vi "DeviceSetNiAuthPasswordRequest_Parse.vi"(8 "error in (no error)":errorcluster, 11 "Message":T5) -> (0 "error out":errorcluster, 1 "Body":T1, 2 "Header":T3, 3 "DeviceSetNiAuthPasswordRequest":T2)   [LabVIEW 2017]
uses:
  <vilib>/addons/InsightCM/MessageBus/Base/controls/Message.ctl
  <vilib>/addons/InsightCM/MessageBus/Base/controls/MessageHeader.ctl
  <vilib>/addons/InsightCM/MessageBus/Base/controls/KeyValuePair.ctl
  <vilib>/addons/InsightCM/MessageBus/MessageLibrary/Device/controls/DeviceSetNiAuthPasswordRequest.ctl
  <vilib>/addons/InsightCM/MessageBus/MessageLibrary/Device/controls/DeviceSetNiAuthPasswordRequestBody.ctl
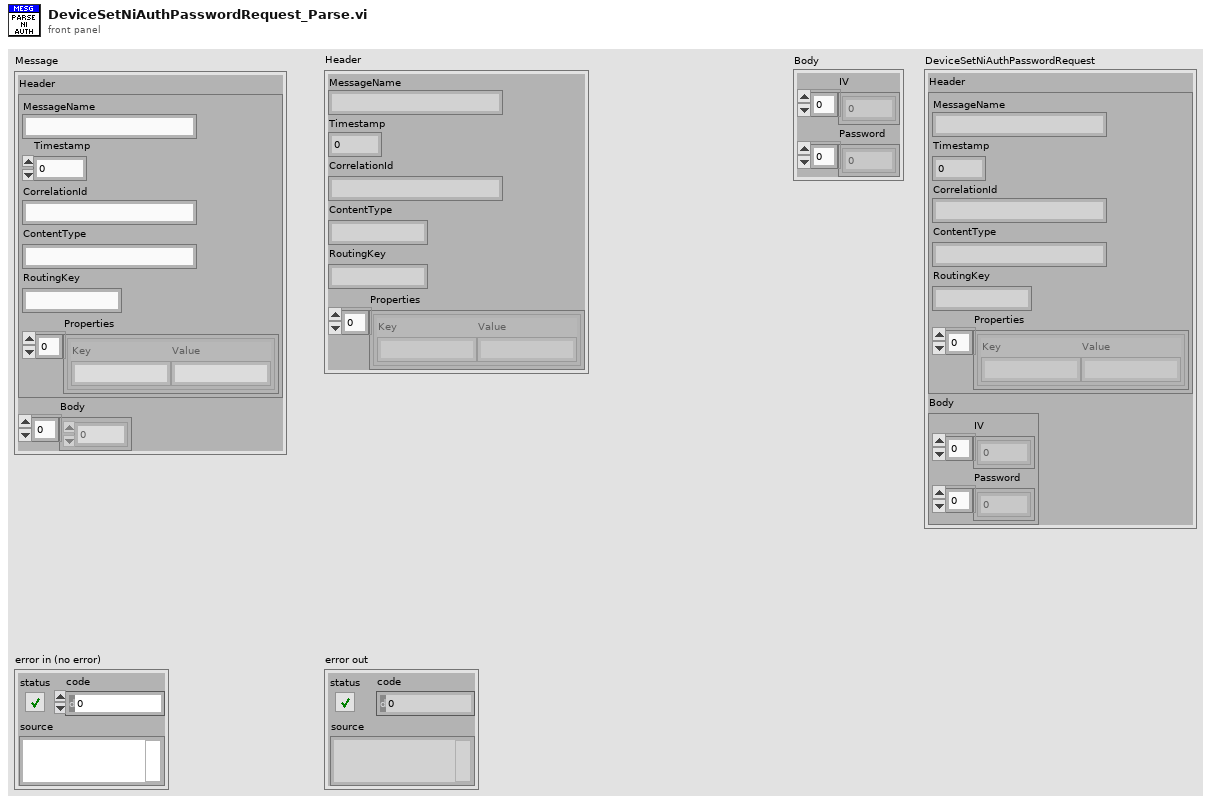
[diagram p1: front panel]
types:
  T1 = typedef "DeviceSetNiAuthPasswordRequestBody.ctl" = cluster{"IV":u8[], "Password":u8[]}
  T2 = typedef "DeviceSetNiAuthPasswordRequest.ctl" = cluster{"Header":T3, "Body":T1}
  T3 = typedef "MessageHeader.ctl" = cluster{"MessageName":string, "Timestamp":i64, "CorrelationId":string, "ContentType":string, "RoutingKey":string, "Properties":T4[]}
  T4 = typedef "KeyValuePair.ctl" = cluster{"Key":string, "Value":string}
  T5 = typedef "Message.ctl" = cluster{"Header":T3, "Body":u8[]}
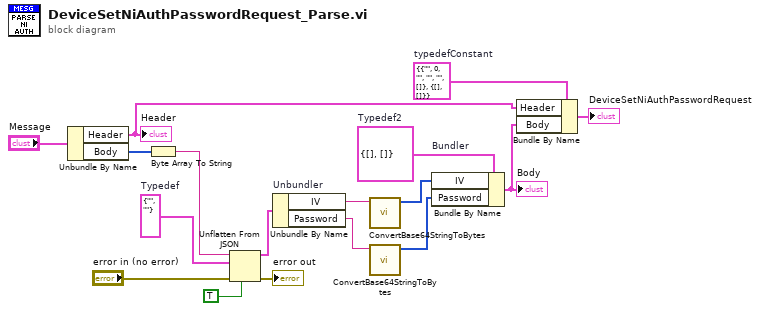
[diagram p0: block diagram]
diagram:
  w5 = T1 {"IV"=[], "Password"=[]}  # Typedef2
  w9 = T2 {"Header"={"MessageName"="", "Timestamp"=0, "CorrelationId"="", "ContentType"="", "RoutingKey"="", "Properties"=[]}, "Body"={"IV"=[], "Password"=[]}}  # typedefConstant
  w13 = cluster{"IV":string, "Password":string} {"IV"="", "Password"=""}  # Typedef
  n1 = Unbundle By Name("Message") -> ("Header"=w15:T3, "Body"=w7:u8[])
  "Header" <- w15
  n2 = Byte Array To String(unsigned byte array=w7) -> (string=w12:string)
  n3 = Unflatten From JSON(JSON string=w12, type and defaults=w13, default null elements? (F)=TRUE, error in (no error)="error in (no error)") -> (value=w11:cluster{"IV":string, "Password":string}, error out=→"error out":errorcluster)  [unwired: 3 in]
  n4 = Unbundle By Name "Unbundler"(w11) -> ("IV"=w4:string, "Password"=w2:string)
  n5 = call <vilib>:"ConvertBase64StringToBytes.vi"("Base64 string"=w4) -> ("U8 array"=w3:u8[])  [unwired: 9 in, 1 out]
  n6 = call <vilib>:"ConvertBase64StringToBytes.vi"("Base64 string"=w2) -> ("U8 array"=w1:u8[])  [unwired: 9 in, 1 out]
  n7 = Bundle By Name "Bundler"(cluster=w5, "IV"=w3, "Password"=w1) -> (w6:T1)
  "Body" <- w6
  n8 = Bundle By Name(cluster=w9, "Header"=w15, "Body"=w6) -> (→"DeviceSetNiAuthPasswordRequest":T2)
